vi "FindNameInTree_test.vi"() -> ()   [LabVIEW 2013]
uses:
  <vilib>/Utility/miscctls.llb/LVSelectionTypeDef.ctl
  VIs_LVTM/FindName Task_Manager Library/FindName Task_Manager.lvlib
panel:
  out "Found/Total =":string
  in  "Data Tree":refnum<vi>
  in  "NameToFind":string caption="Find ="
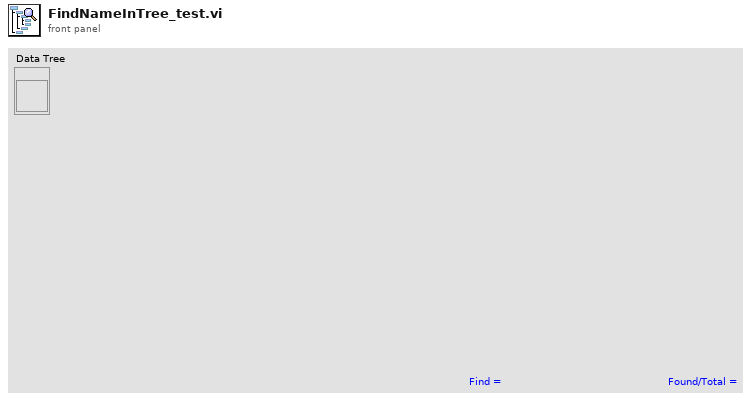
[diagram p1: front panel]
types:
  T1 = typedef "LVSelectionTypeDef.ctl" = cluster{"Selection Start":u32, "Selection End":u32}
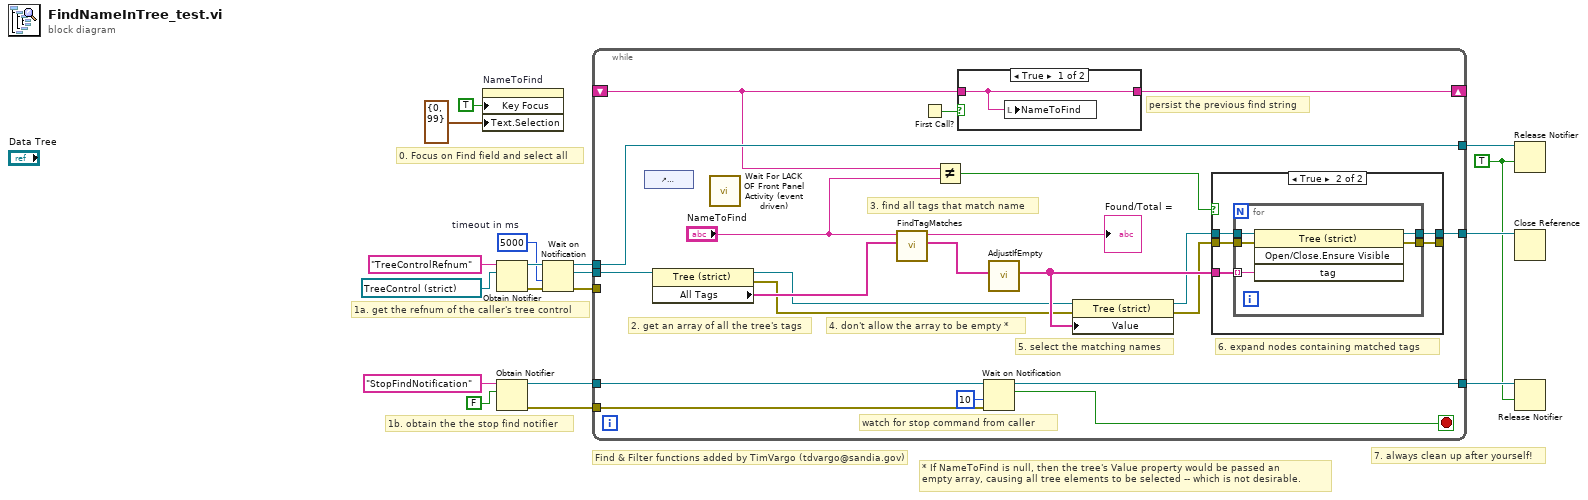
[diagram p0: block diagram]
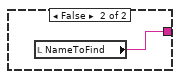
[diagram p3: hidden frame]
diagram:
  w1 = TRUE ("force destroy? (F)")
  w5 = 5000  # timeout in ms
  # "Find & Filter functions added by TimVargo (tdvargo@sandia.gov)"
  # "* If NameToFind is null, then the tree's Value property would be passed an \nempty array, causing all tree elements to be selected -- which is not desirable."
  # "1b. obtain the the stop find notifier"
  # "0. Focus on Find field and select all"
  # "7. always clean up after yourself!"
  # "1a. get the refnum of the caller's tree control"
  n1 = property on="NameToFind" class="Str"("Key Focus"=TRUE, "Text.Selection"=T1 {"Selection Start"=0, "Selection End"=99}) -> ()  [unwired: 2 in, 2 out]
  n2 = Obtain Notifier(name (unnamed)="TreeControlRefnum", notification data type=refnum<vi> refnum ("Data Tree")) -> (notifier out=w15:refnum<notifier>, error out=w16:errorcluster)  [unwired: 2 in, 1 out]
  n3 = Obtain Notifier(name (unnamed)="StopFindNotification", notification data type=FALSE) -> (notifier out=w4:refnum<notifier>, error out=w3:errorcluster)  [unwired: 2 in, 1 out]
  n4 = Wait on Notification(notifier=w15, timeout in ms (-1)=w5, error in (no error)=w16) -> (notifier out=w13:refnum<notifier>, notification=w14:refnum<vi>, error out=w10:errorcluster)  [unwired: 1 in, 1 out]
  n5 = while {
    tunnel: w14 -> [w38]
    tunnel: w13 -> [w37]
    tunnel: [w37] -> w12
    tunnel: [w22] -> w11
    tunnel: w10 -> [_]
    shift-right: [w34] -> _
    shift-left: _ -> [w19]
    tunnel: w4 -> [w32]
    tunnel: w3 -> [w31]
    tunnel: [w30] -> w2
    stop <- w27 stop-if-true
    # "6. expand nodes containing matched tags"
    # "4. don't allow the array to be empty *"
    # "watch for stop command from caller"
    # "persist the previous find string"
    # "3. find all tags that match name"
    # "5. select the matching names"
    # "2. get an array of all the tree's tags"
    n6 = control-ref of="NameToFind"() -> ()  [unwired: 1 out]
    n7 = property class="Tree (strict)"(reference=w38) -> (reference out=w20:refnum<vi>, error out=w21:errorcluster, "All Tags"=w33:string[])  [unwired: 1 in]
    n8 = call "Wait For LACK OF Front Panel Activity (event driven).vi"() -> ()  [unwired: 10 in, 1 out]
    n9 = call "FindTagMatches.vi"("All Tags"=w33, "NameToFind"="NameToFind") -> ("Found"=w36:string[], "ResultString"=→"Found/Total =":string)  [unwired: 7 in, 1 out]
    n10 = First Call?() -> (First Call?: T/F=w35:bool)
    n11 = Not Equal?(x=w19, y="NameToFind") -> (x != y?=w25:bool)
    n12 = case shown="True" w35 {
      tunnel: [w52 w53] -> w34
      tunnel: w19 -> [w52 _]
      frame True {
        n13 = local write "NameToFind"(w52) -> ()
      }
      frame False {
        n14 = local read "NameToFind"() -> (w53:string)
      }
    }
    n15 = Wait on Notification(notifier=w32, timeout in ms (-1)=10, error in (no error)=w31) -> (notifier out=w30:refnum<notifier>, notification=w27:bool)  [unwired: 1 in, 2 out]
    n16 = call "AdjustIfEmpty.vi"("Found"=w36) -> ("FoundAdj"=w28:string[])  [unwired: 10 in]
    n17 = property class="Tree (strict)"(reference=w20, error in=w21, "Value"=w28) -> (reference out=w24:refnum<vi>, error out=w23:errorcluster)
    n18 = case shown="True" w25 {
      tunnel: [w40 w46] -> _
      tunnel: w23 -> [w40 w45]
      tunnel: w24 -> [w41 w44]
      tunnel: [w41 w43] -> w22
      tunnel: w28 -> [_ w42]
      frame False {
      }
      frame True {
        n19 = for {
          tunnel: [w51] -> w46
          tunnel: w45 -> [w50]
          tunnel: w44 -> [w49]
          tunnel: [w48] -> w43
          tunnel: w42 -> [w47] mode=indexing
          n20 = invoke class="Tree (strict)" method="Open/Close.Ensure Visible"(reference=w49, error in=w50, "tag"=w47) -> (reference out=w48:refnum<vi>, error out=w51:errorcluster)  [unwired: 1 in, 2 out]
        }
      }
    }
  }
  n21 = Release Notifier(notifier=w12, force destroy? (F)=w1) -> ()  [unwired: 1 in, 3 out]
  n22 = Close Reference(reference=w11) -> ()  [unwired: 1 in, 1 out]
  n23 = Release Notifier(notifier=w2, force destroy? (F)=w1) -> ()  [unwired: 1 in, 3 out]
